vi "PageExplorer_Global_Init.vi"(11 "Object":T1) -> ()   [LabVIEW 2020]
uses:
  <resource>/Framework/Providers/API/ItemRef.ctl
  <resource>/dialog/lvconfig.llb/LV Config Read Boolean.vi
panel:
  out "error out":errorcluster
  in  "error in":errorcluster
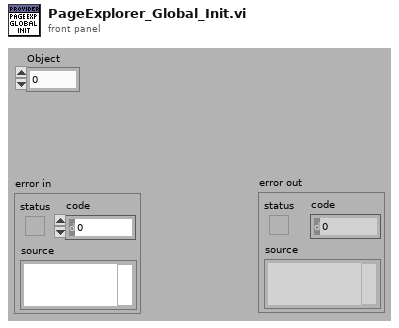
[diagram p1: front panel]
types:
  T1 = typedef "ItemRef.ctl" = u64
  T2 = enum32{"Invalid", "Standard", "Closed", "Hidden", "Minimized", "Maximized"}
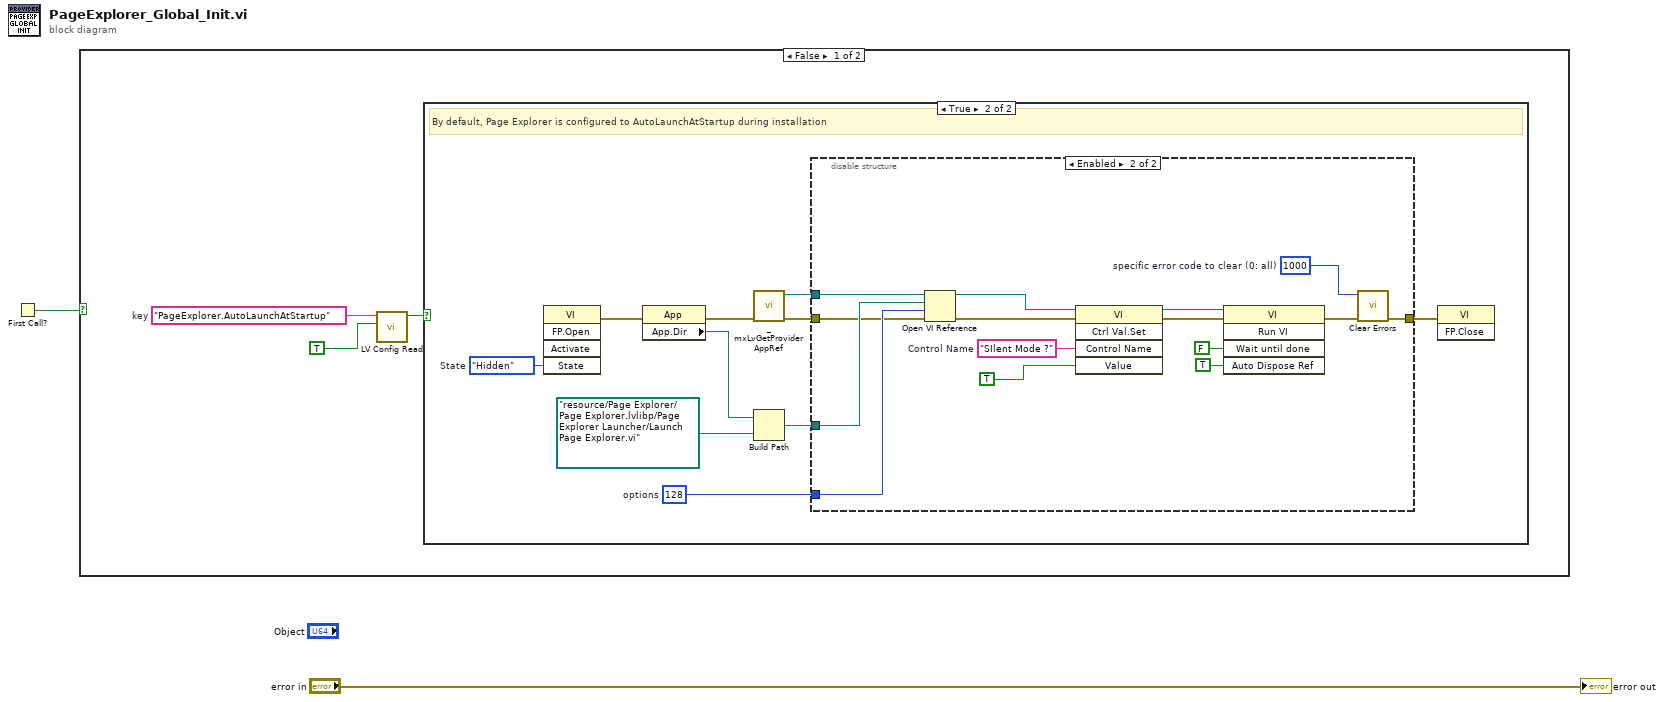
[diagram p0: block diagram]
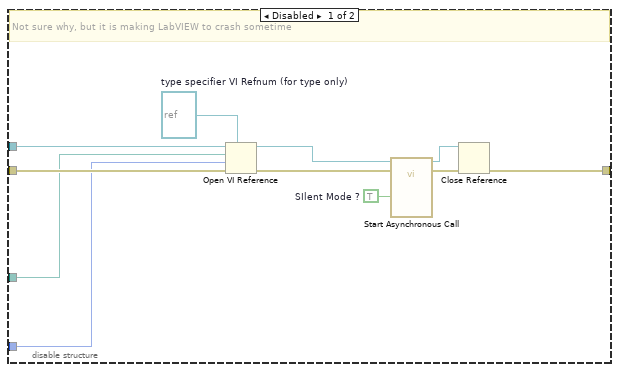
[diagram p3: hidden frame]
diagram:
  n1 = First Call?() -> (First Call?: T/F=w1:bool)
  n2 = case shown="False" w1 {
    frame False {
      w5 = "PageExplorer.AutoLaunchAtStartup"  # key
      n3 = call-poly <resource>:"LV Config Read.vi"("default value"=TRUE, "key"=w5) -> ("value"=w3:bool)  [unwired: 3 in, 2 out]
      n4 = case shown="True" w3 {
        frame False {
        }
        frame True {
          w9 = 128  # options
          w15 = T2."Hidden"  # State
          # "By default, Page Explorer is configured to AutoLaunchAtStartup during installation"
          n5 = invoke class="VI" method="FP.Open"("State"=w15) -> (error out=w12:errorcluster)  [unwired: 4 in, 4 out]
          n6 = property class="App"(error in=w12) -> (error out=w11:errorcluster, "App.Dir"=w14:path)  [unwired: 1 in, 1 out]
          n7 = call "_mxLvGetProviderAppRef.vi"("error in"=w11) -> ("error out"=w6:errorcluster, "App Reference"=w7:refnum<vi>)  [unwired: 9 in]
          n8 = Build Path(base path=w14, name or relative path=path "resource/Page Explorer/Page Explorer.lvlibp/Page Explorer Launcher/Launch Page Explorer.vi" ("vi path")) -> (appended path=w8:path)
          n9 = disable-structure shown="Enabled" {
            disable-tunnel: w6 -> [w22 w30]
            disable-tunnel: [w24 w28] -> w10
            disable-tunnel: w9 -> [w16 w34]
            disable-tunnel: w8 -> [w17 w33]
            disable-tunnel: w7 -> [w18 w32]
            frame Disabled {
              w20 = refnum<vi> refnum  # type specifier VI Refnum (for type only)
              w25 = TRUE  # SIlent Mode ?
              # "Not sure why, but it is making LabVIEW to crash sometime"
              n10 = Open VI Reference(type specifier VI Refnum (for type only)=w20, application reference (local)=w18, vi path=w17, options=w16, error in (no error)=w22) -> (vi reference=w19:refnum<vi>, error out=w21:errorcluster)  [unwired: 1 in]
              n11 = call-by-ref "Start Asynchronous Call"(reference=w19, error in=w21, "SIlent Mode ?"=w25) -> (reference out=w23:refnum<vi>, error out=w26:errorcluster)
              n12 = Close Reference(reference=w23, error in (no error)=w26) -> (error out=w24:errorcluster)
            }
            frame Enabled {
              w27 = 1000  # specific error code to clear (0: all)
              w36 = "SIlent Mode ?"  # Control Name
              n13 = Open VI Reference(application reference (local)=w32, vi path=w33, options=w34, error in (no error)=w30) -> (vi reference=w31:refnum<vi>, error out=w29:errorcluster)  [unwired: 2 in]
              n14 = invoke class="VI" method="Ctrl Val.Set"(reference=w31, error in=w29, "Control Name"=w36, "Value"=TRUE ("Auto Dispose Reference")) -> (reference out=w37:refnum<vi>, error out=w38:errorcluster)  [unwired: 1 in, 3 out]
              n15 = invoke class="VI" method="Run VI"(reference=w37, error in=w38, "Wait until done"=FALSE ("Wait Until Done"), "Auto Dispose Ref"=TRUE ("Auto Dispose Reference")) -> (error out=w39:errorcluster)  [unwired: 1 in, 4 out]
              n16 = call <vilib>:"Clear Errors.vi"("error in (no error)"=w39, "specific error code to clear (0: all)"=w27) -> ("error out"=w28:errorcluster)  [unwired: 4 in, 1 out]
            }
          }
          n17 = invoke class="VI" method="FP.Close"(error in=w10) -> ()  [unwired: 2 in, 3 out]
        }
      }
    }
    frame True {
      # "Don't Launch the tool when LabVIEW Launches, instead Launch it when a Project is Loading"
    }
  }
  "error out" <- "error in"
